vi "Eagle_FPGA Scanner Control_1.vi"() -> ()   [LabVIEW 2015]
uses:
  <vilib>/Platform/TimedLoop/XDataNode/timing_clust.ctl
  <vilib>/Platform/TimedLoop/XDataNode/nitl_modes.ctl
  <vilib>/Platform/TimedLoop/XDataNode/wakeup.ctl
  <vilib>/rvi/Emulation/niFpgaGetClockAttributes.vi
  <vilib>/rvi/Emulation/niFpgaSctlEmulationGetInTimedLoop.vi
  <vilib>/rvi/Emulation/niFpgaEmulationReportErrorSimple.vi
  <vilib>/rvi/Emulation/niFpgaProcessEmulError.vi
  <vilib>/rvi/eio/common/nirviEmuTemplateMethod_errors.vi
  <vilib>/rvi/Emulation/niFpgaCriticalErrorInLSC.vi
  <vilib>/rvi/FXPMathLib/FxpAdd/XNode/nifxpmath_Add.xnode
  <vilib>/rvi/FXPMathLib/FxpMul/XNode/nifxpmath_Multiplier.xnode
  <vilib>/eio/EIONode/EIONode.xnode
  <vilib>/Platform/TimedLoop/XDataNode/XDataNode.xnode
  <vilib>/rvi/FXPMathLib/sim/FxpSim.dll
  <vilib>/Platform/TimedLoop/XDataNode/XDNodeRunTimeDep.lvlib
panel:
  in  "PY":fxp<+,10,10>
  in  "PX":fxp<+,10,10>
  in  "NoGO Zone":T1
  in  "Center":cluster{"CX":fxp<+,10,10>, "CY":fxp<+,10,10>}
  in  "NumOfRetries":u16
  out "VX CMD":fxp<+/-,20,5>
  out "VY CMD":fxp<+/-,20,5>
  out "SCAN ENA":bool
  in  "VY OFFS":fxp<+/-,16,1>
  in  "VX OFFS":fxp<+/-,16,1>
  in  "Reset":bool
  out "Y CMD IND":fxp<+/-,20,5>
  out "X CMD IND":fxp<+/-,20,5>
  out "Mod3/AI1":fxp<+,18,3>
  out "Mod3/AI0":fxp<+,18,3>
  in  "Mod3/AO1":fxp<+,16,3>
  in  "Mod3/AO0":fxp<+,16,3>
  out "Y READ":fxp<+/-,20,5>
  out "X READ":fxp<+/-,20,5>
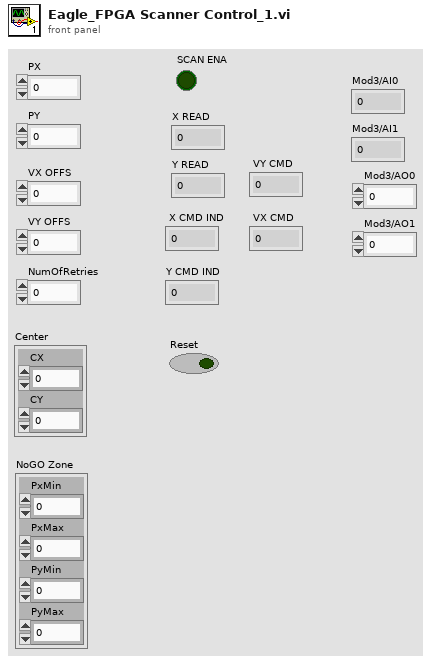
[diagram p1: front panel]
types:
  T1 = cluster{"PxMin":fxp<+,10,10>, "PxMax":fxp<+,10,10>, "PyMin":fxp<+,10,10>, "PyMax":fxp<+,10,10>}
  T2 = typedef "XDNodeRunTimeDep.lvlib/timing_clust.ctl" = cluster{"Expected End [f-1]":u64, "Actual End [f-1]":u64, "Finished Late? [f-1]":bool, "Expected End [i-1]":u64, "Actual End [i-1]":u64, "Finished Late? [i-1]":bool, "Expected Start [i]":u64, "Actual Start [i]":u64, "Expected Start [f]":u64, "Actual Start [f]":u64, "Source Name":string, "Structure Name":string, "Period":i64, "Deadline":i64, "Offset":i64, "Start":i64, "Priority":i32, "Timeout":i32, "Mode":T3, "Wakeup Reason":T4, "Error":errorcluster, "Source Type":string, "Secondary Source Type":string, "Global End Time":u64, "Global Start Time":u64, "Frame Duration":u64, "Iteration Duration":u64, "Assigned CPU":i32, "I/O Scan Engine Mode":u32}
  T3 = typedef "XDNodeRunTimeDep.lvlib/nitl_modes.ctl" = enum32{"No Change", "Process missed periods, maintain original phase", "Discard missed periods, maintain original phase", "Process missed periods, ignore original phase", "Discard missed periods, ignore original phase"}
  T4 = typedef "XDNodeRunTimeDep.lvlib/wakeup.ctl" = enum32{"Normal", "Aborted", "Asynchronous wakeup", "Timing source error", "Timed loop error", "Timeout"}
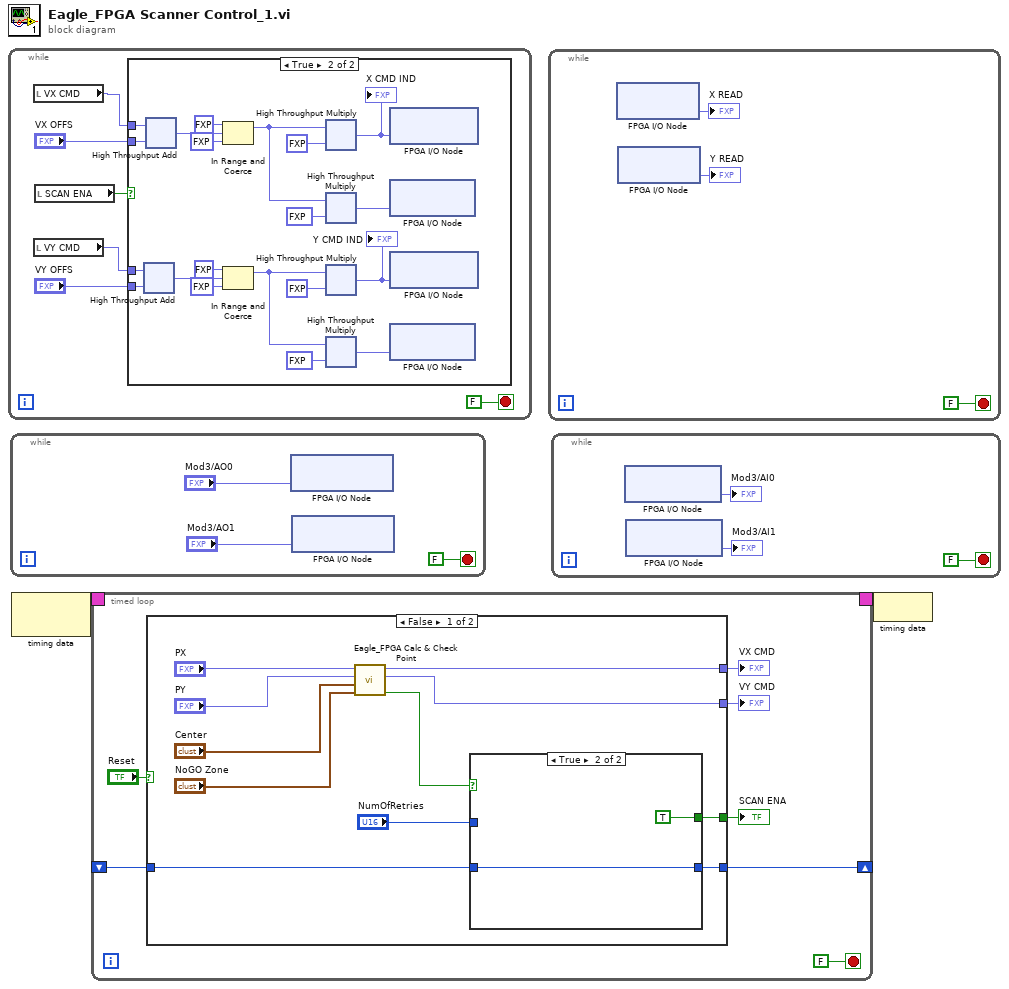
[diagram p0: block diagram]
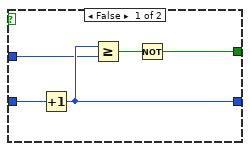
[diagram p2: hidden frame]
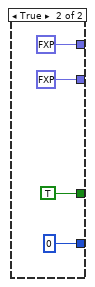
[diagram p3: hidden frame]
diagram:
  n1 = while {
    stop <- FALSE stop-if-true
    n2 = local read "VX CMD"() -> (w4:fxp<+/-,20,5>)
    n3 = local read "VY CMD"() -> (w3:fxp<+/-,20,5>)
    n4 = local read "SCAN ENA"() -> (w5:bool)
    n5 = case shown="True" w5 {
      tunnel: "VX OFFS" -> [_ w20]
      tunnel: "VY OFFS" -> [_ w19]
      tunnel: w4 -> [_ w10]
      tunnel: w3 -> [_ w9]
      frame False {
      }
      frame True {
        n6 = xnode "High Throughput Add"("x"=w9, "y"=w19) -> ("x+y"=w12:fxp<+/-,21,6>)
        n7 = xnode "High Throughput Add"("x"=w10, "y"=w20) -> ("x+y"=w18:fxp<+/-,21,6>)
        n8 = In Range and Coerce(upper limit=fxp<+/-,20,5> 10.0, x=w18, lower limit=fxp<+/-,20,5> -10.0 ("upper limit")) -> (coerced(x)=w17:fxp<+/-,21,6>)  [unwired: 1 out]
        n9 = In Range and Coerce(upper limit=fxp<+/-,20,5> 10.0, x=w12, lower limit=fxp<+/-,20,5> -10.0 ("upper limit")) -> (coerced(x)=w11:fxp<+/-,21,6>)  [unwired: 1 out]
        n10 = xnode ("High Throughput Multiply")("x"=w17, "y"=fxp<+/-,20,5> 0.5) -> ("x*y"=w26:fxp<+/-,20,5>)
        "X CMD IND" <- w26
        n11 = xnode ("High Throughput Multiply")("x"=w17, "y"=fxp<+/-,20,5> -0.5) -> ("x*y"=w24:fxp<+/-,20,5>)
        n12 = xnode ("High Throughput Multiply")("x"=w11, "y"=fxp<+/-,20,5> 0.5) -> ("x*y"=w22:fxp<+/-,20,5>)
        "Y CMD IND" <- w22
        n13 = xnode ("High Throughput Multiply")("x"=w11, "y"=fxp<+/-,20,5> -0.5) -> ("x*y"=w21:fxp<+/-,20,5>)
        n14 = xnode "FPGA I/O Node"("X CMD+"=w26) -> ()  [unwired: 1 in, 1 out]
        n15 = xnode "FPGA I/O Node"("X CMD-"=w24) -> ()  [unwired: 1 in, 1 out]
        n16 = xnode "FPGA I/O Node"("Y CMD+"=w22) -> ()  [unwired: 1 in, 1 out]
        n17 = xnode "FPGA I/O Node"("Y CMD-"=w21) -> ()  [unwired: 1 in, 1 out]
      }
    }
  }
  n18 = while {
    stop <- FALSE stop-if-true
    n19 = xnode "FPGA I/O Node"("Mod3/AO0"="Mod3/AO0") -> ()  [unwired: 1 in, 1 out]
    n20 = xnode "FPGA I/O Node"("Mod3/AO1"="Mod3/AO1") -> ()  [unwired: 1 in, 1 out]
  }
  n21 = node-c288() -> (w2:T2)  [unwired: 1 in]
  n22 = timed-loop {
    timing: w2 -> [_]
    timing-out: [_] -> w1
    shift-right: [w33] -> _
    shift-left: _ -> [w32]
    stop <- FALSE stop-if-true
    n23 = case shown="False" "Reset" {
      tunnel: [w49 fxp<+/-,20,5> 10.0 ("VX CMD")] -> w36
      tunnel: [w48 fxp<+/-,20,5> 10.0 ("VY CMD")] -> w35
      tunnel: [w43 TRUE ("SCAN ENA")] -> w34
      tunnel: [w45 u16 0] -> w33
      tunnel: w32 -> [w46 _]
      frame False {
        n24 = call "Eagle_FPGA Calc & Check Point.vi"("NoGO Zone"="NoGO Zone", "Center"="Center", "PX"="PY", "PY"="PX") -> ("SCAN ENA"=w47:bool, "VY CMD"=w48:fxp<+/-,20,5>, "VX CMD"=w49:fxp<+/-,20,5>)  [unwired: 5 in]
        n25 = case shown="True" w47 {
          tunnel: w46 -> [w54 w55]
          tunnel: [w53 w55] -> w45
          tunnel: "NumOfRetries" -> [w52 _]
          tunnel: [w50 TRUE] -> w43
          frame False {
            n26 = Increment(x=w54) -> (x+1=w53:u16)
            n27 = Greater Or Equal?(x=w53, y=w52) -> (x >= y?=w51:bool)
            n28 = Not(x=w51) -> (.not. x?=w50:bool)
          }
          frame True {
          }
        }
      }
      frame True {
      }
    }
    "SCAN ENA" <- w34
    "VY CMD" <- w35
    "VX CMD" <- w36
  }
  n29 = while {
    stop <- FALSE stop-if-true
    n30 = xnode "FPGA I/O Node"() -> ("X READ"=→"X READ":fxp<+/-,20,5>)  [unwired: 1 in, 1 out]
    n31 = xnode "FPGA I/O Node"() -> ("Y READ"=→"Y READ":fxp<+/-,20,5>)  [unwired: 1 in, 1 out]
  }
  n32 = while {
    stop <- FALSE stop-if-true
    n33 = xnode "FPGA I/O Node"() -> ("Mod3/AI0"=→"Mod3/AI0":fxp<+,18,3>)  [unwired: 1 in, 1 out]
    n34 = xnode "FPGA I/O Node"() -> ("Mod3/AI1"=→"Mod3/AI1":fxp<+,18,3>)  [unwired: 1 in, 1 out]
  }
  n35 = node-c288(w1) -> ()
